vi "dvm Get Single.vi"(8 "error in (no error)":errorcluster, 11 "dvm session in":T2) -> (0 "error out":errorcluster, 2 "reading":T1, 3 "dvm session out":T2)   [LabVIEW 2020]
doc: "Close auxiliary DVM."
uses:
  dvm session.ctl
  dvm type.ctl
  drivers/Fluke 5790A/top_level/F5790 session.ctl
  dvm Reading.ctl
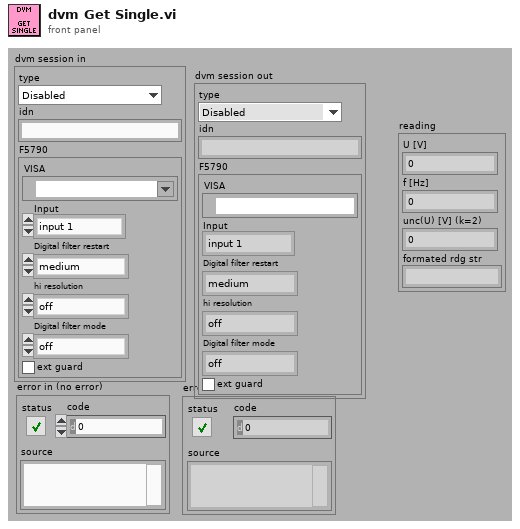
[diagram p1: front panel]
types:
  T1 = typedef "dvm Reading.ctl" = cluster{"U [V]":dbl, "f [Hz]":dbl, "unc(U) [V] (k=2)":dbl, "formated rdg str":string}
  T2 = typedef "dvm session.ctl" = cluster{"type":T3, "idn":string, "F5790":T4}
  T3 = typedef "dvm type.ctl" = enum16{"Disabled", "Simulated", "Fluke 5790A"}
  T4 = typedef "F5790 session.ctl" = cluster{"VISA":refnum<visa-resource-name>, "Input":enum16{"input 1", "input 2", "wide-band"}, "Digital filter restart":enum16{"medium", "fine", "coarse"}, "hi resolution":enum16{"off", "on"}, "Digital filter mode":enum16{"off", "fast", "medium", "slow"}, "ext guard":bool}
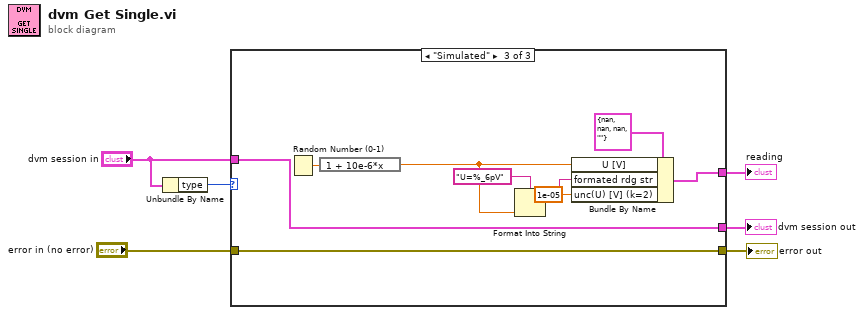
[diagram p0: block diagram]
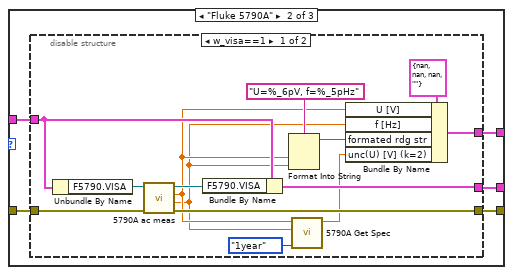
[diagram p3: hidden frame]
diagram:
  n1 = Unbundle By Name("dvm session in") -> ("type"=w6:T3)
  n2 = case shown="\"Simulated\"" w6 {
    tunnel: "dvm session in" -> [w7 w12 w37]
    tunnel: "error in (no error)" -> [w8 w13 w38]
    tunnel: [w8 w11 w38] -> w3
    tunnel: [w7 w10 w37] -> w2
    tunnel: [_ w9 w31] -> w1
    frame "Disabled", Default {
    }
    frame "Fluke 5790A" {
      n3 = disable-structure shown="w_visa==1" {
        disable-tunnel: w13 -> [w27 w29]
        disable-tunnel: w12 -> [w24 w28]
        disable-tunnel: [w25 w29] -> w11
        disable-tunnel: [w22 w28] -> w10
        disable-tunnel: [w18 _] -> w9
        frame condition #0 (active) {
          n4 = Unbundle By Name(w24) -> ("F5790.VISA"=w26:refnum<visa-resource-name>)
          n5 = call "5790A ac meas.vi"("error in"=w27, "5790A"=w26) -> ("error out"=w25:errorcluster, "Frequency"=w16:dbl, "Voltage"=w17:dbl, "Session Out"=w23:refnum<visa-resource-name>)  [unwired: 2 in, 2 out]
          n6 = Bundle By Name(cluster=w24, "F5790.VISA"=w23) -> (w22:T2)
          n7 = Format Into String(format string="U=%_6pV, f=%_5pHz", w17, w16) -> (resulting string=w20:string)  [unwired: 2 in, 1 out]
          n8 = call "5790A Get Spec.vi"("period"=enum16{"90day", "1year", "2year"}."1year", "f [Hz]"=w16, "U [V]"=w17) -> ("abs unc(U) [V]"=w14:dbl)  [unwired: 7 in, 1 out]
          n9 = Bundle By Name(cluster=T1 {"U [V]"=nan, "f [Hz]"=nan, "unc(U) [V] (k=2)"=nan, "formated rdg str"=""} ("reading"), "U [V]"=w17, "f [Hz]"=w16, "formated rdg str"=w20, "unc(U) [V] (k=2)"=w14) -> (w18:T1)
        }
        frame condition #1 {
        }
      }
    }
    frame "Simulated" {
      n10 = Random Number (0-1)() -> (number: 0 to 1=w36:dbl)
      n11 = expression code="1 + 10e-6*x"(w36) -> (w33:dbl)
      n12 = Format Into String(format string="U=%_6pV", w33) -> (resulting string=w34:string)  [unwired: 2 in, 1 out]
      n13 = Bundle By Name(cluster=T1 {"U [V]"=nan, "f [Hz]"=nan, "unc(U) [V] (k=2)"=nan, "formated rdg str"=""} ("reading"), "U [V]"=w33, "formated rdg str"=w34, "unc(U) [V] (k=2)"=1e-05) -> (w31:T1)
    }
  }
  "error out" <- w3
  "dvm session out" <- w2
  "reading" <- w1
